vi "lidar_array.vi"(0 "LiDAR Configuration":string="{\n\t\"type\": \"LidarArray\",\n\t\"listen_port\": 6699,\n\t\"location\": {\n\t\t\"x\": 150.0,\n\t\t\"y\": 0.0,\n\t\t\"z\": 60.0\n\t},\n\t\"rotation\": {\n\t\t\"pitch\": 0.0,\n\t\t\"roll\": 0.0,\n\t\t\"yaw\": 0.0\n\t},\n\t\"udp_streamer\": {\n\t\t\"destination_ip\": \"127.0.0.1\",\n\t\t\"udp_packetizer\": \"RSM1\",\n\t\t\"use_udp_streaming\": true\n\t},\n\t\"num_threads\": 10,\n\t\"receive_stream\": false,\n\t\"enable_streaming\": true,\n\t\"firing_data_file_path\":\"\",\n\t\"beam_divergence_horizontal\": 0.009999999776482582,\n\t\"beam_divergence_vertical\": 0.009999999776482582,\n\t\"beam_size_horizontal\": 1.0,\n\t\"beam_size_vertical\": 1.0,\n\t\"debug_draw\": false,\n\t\"diffuse_gain\": 1.0,\n\t\"distance_error\": 1.0,\n\t\"dropout_threshold\": 0.0,\n\t\"intensity_error\": 0.05000000074505806,\n\t\"max_distance\": 150000.0,\n\t\"post_gain\": 1.0,\n\t\"specular_gain\": 1.0,\n\t\"wait_for_fresh_frame\": true,\n\t\"wind_effect\": 0.0\n}", 3 "error in":errorcluster={"status"=FALSE, "code"=0, "source"="\"complete\","}) -> (4 "LiDAR Configuration":string="{\n    \"type\": \"LidarArray\",\n    \"packet_size\": 1472,\n    \"listen_port\": 8201,\n    \"synchronized_display\": true,\n    \"location\": {\n      \"x\": 150.0,\n      \"y\": 0.0,\n      \"z\": 190.0\n    },\n    \"rotation\": {\n      \"pitch\": 0.0,\n      \"yaw\": 0.0,\n      \"roll\": 0.0\n    },\n    \"max_distance\": 10000.0,\n    \"beam_divergence_horizontal\": 0.01,\n    \"beam_divergence_vertical\": 0.01,\n    \"beam_size_horizontal\": 1.0,\n    \"beam_size_vertical\": 1.0,\n    \"distance_error\": 0.075,\n    \"num_threads\": 6,\n    \"intensity_error\": 0.1,\n    \"debug_draw\": false,\n    \"lidar_model\": 0,\n    \"specular_gain\": 1.25,\n    \"diffuse_gain\": 0.95,\n    \"post_gain\": 1.15\n}", 5 "LiDAR Data":T1(array[cluster]), 6 "Raw data":string, 7 "error out":errorcluster={"status"=FALSE, "code"=0, "source"="\"complete\","})   [LabVIEW 2019, in "Lib_Simx.lvlib"]
doc: "Configure and process the data stream for an array LiDAR sensor."
uses:
  Lib_Simx.lvlib
  tools/simx_common.vi
  controls/Header.ctl
panel:
  out "Header":T2
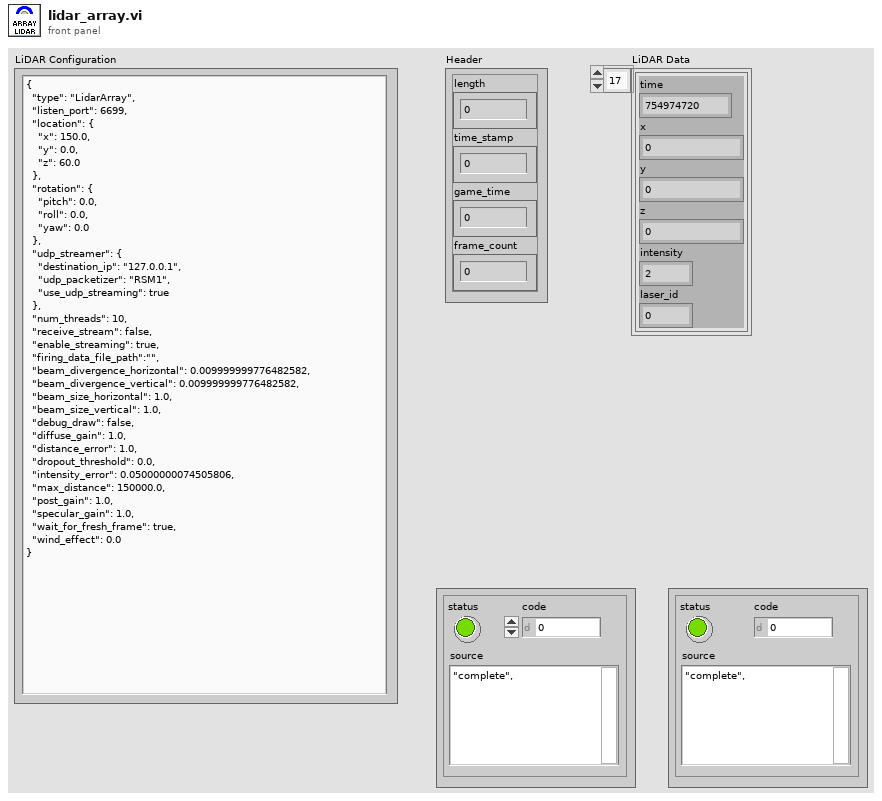
[diagram p1: front panel]
types:
  T1 = cluster{"time":u32, "x":sgl, "y":sgl, "z":sgl, "intensity":u8, "laser_id":u8}[]
  T2 = typedef "Lib_Simx.lvlib/Header.ctl" = cluster{"length":u32, "time_stamp":u32, "game_time":sgl, "frame_count":u32}
  T3 = enum16{"big-endian, network order", "native, host order", "little-endian"}
  T4 = typedef "Lib_Simx.lvlib/sensor_sample.ctl" = cluster{"Header":T2, "data out":string}
  T5 = typedef "Lib_Simx.lvlib/simx_connection.ctl" = cluster{"Config":T6, "Connections":T9, "Map":cluster{"lanes":cluster{"x":dbl[], "y":dbl[], "z":dbl[]}, "StartPosition":cluster{"start_points":T10, "StartRotation":dbl[], "StartLocation":dbl[]}, "Draw Map Size":T11, "DrawArea":cluster{"min_Y":dbl, "min_X":dbl, "Scale X":dbl, "Scale Y":dbl}, "Map":picture, "Map Geojson":string}}
  T6 = typedef "Lib_Simx.lvlib/config.ctl" = cluster{"Trajectory":T7, "Weather":T8}
  T7 = typedef "Lib_Simx.lvlib/trajectory.ctl" = cluster{"Number of frames":i32, "Frame number":i32, "Trajectory":string}
  T8 = typedef "Lib_Simx.lvlib/weather.ctl" = cluster{"id":string}
  T9 = typedef "Lib_Simx.lvlib/connections.ctl" = cluster{"Simulator Connection":refnum<k5>, "server_ip":string, "Port":i32, "Sensor connections":refnum<k5>[]}
  T10 = typedef "Lib_Simx.lvlib/start_points.ctl" = cluster{"locations":dbl[][], "rotations":dbl[][], "type":string[]}
  T11 = typedef "LVBoundsTypeDef.ctl" = cluster{"Width":u32, "Height":u32}
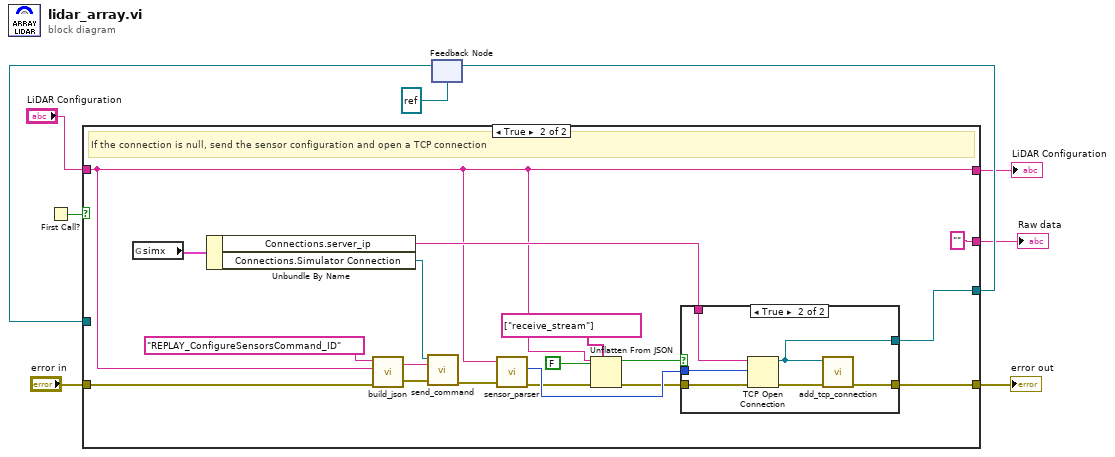
[diagram p0: block diagram]
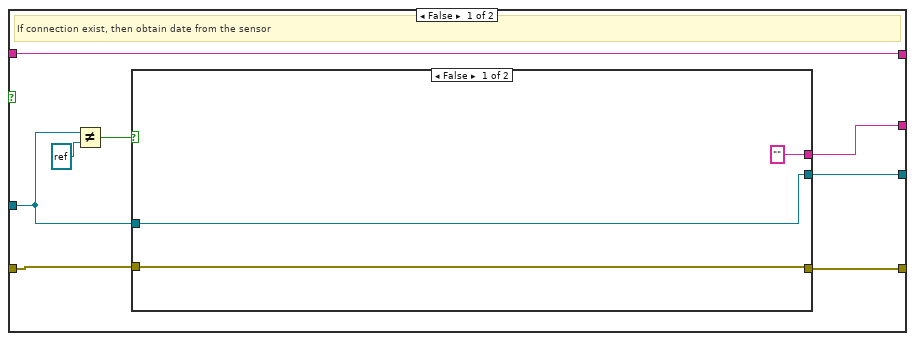
[diagram p2: hidden frame]
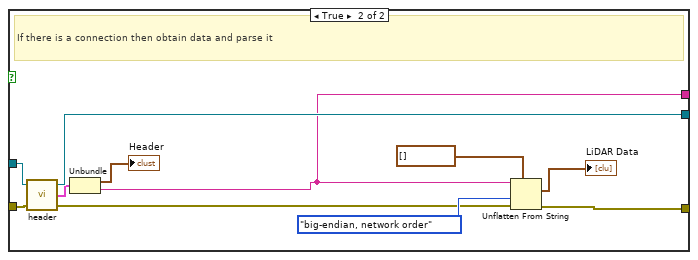
[diagram p3: hidden frame]
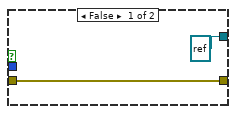
[diagram p4: hidden frame]
diagram:
  n1 = First Call?() -> (First Call?: T/F=w1:bool)
  n2 = feedback #1(refnum<k5> refnum ("lidar_connection")) -> (w5:refnum<k5>)
  n3 = case shown="True" w1 {
    tunnel: [w14 w39] -> w9
    tunnel: "LiDAR Configuration" -> [w15 w36]
    tunnel: [w17 w38] -> w7
    tunnel: w5 -> [w12 _]
    tunnel: "error in" -> [w16 w46]
    tunnel: [w15 w36] -> w3
    tunnel: [w13 "" ("data out")] -> w2
    frame False {
      # "If connection exist, then obtain date from the sensor"
      n4 = Not Equal?(x=w12, y=refnum<k5> refnum) -> (x != y?=w10:bool)
      n5 = case shown="False" w10 {
        tunnel: [w19 w31] -> w17
        tunnel: w16 -> [w20 w30]
        tunnel: [w20 w29] -> w14
        tunnel: ["" ("data out") w28] -> w13
        tunnel: w12 -> [w19 w27]
        frame False {
        }
        frame True {
          # "If there is a connection then obtain data and parse it"
          n6 = call "header.vi"("error in"=w30, "TCP Network Connection in"=w27) -> ("error out"=w22:errorcluster, "Sensor sample"=w26:T4, "TCP Network Connection out"=w31:refnum<k5>)  [unwired: 1 in]
          n7 = Unbundle(w26) -> ("Header"=→"Header":T2, "data out"=w28:string)
          n8 = Unflatten From String(type=T1 [] ("rsm1 format"), binary string=w28, byte order (0:big-endian, network order)=T3."big-endian, network order", error in (no error)=w22) -> (value=→"LiDAR Data":T1, error out=w29:errorcluster)  [unwired: 1 in, 1 out]
        }
      }
    }
    frame True {
      # "If the connection is null, send the sensor configuration and open a TCP connection"
      n9 = global read "simx_common.vi" "simx"() -> (w44:T5)
      n10 = Unbundle By Name(w44) -> ("Connections.server_ip"=w40:string, "Connections.Simulator Connection"=w45:refnum<k5>)
      n11 = call "build_json.vi"("error in"=w46, "Message"=w36, "Command_ID"="REPLAY_ConfigureSensorsCommand_ID") -> ("error out"=w47:errorcluster, "JSON Out"=w48:string)  [unwired: 1 in]
      n12 = call "send_command.vi"("error in"=w47, "JSON Command"=w48, "TCP Network Connection in"=w45) -> ("error out"=w41:errorcluster)  [unwired: 1 in, 3 out]
      n13 = call "sensor_parser.vi"("Sensor configuration"=w36, "error in"=w41) -> ("Port out"=w42:u16, "error out"=w33:errorcluster)  [unwired: 1 in, 2 out]
      n14 = Unflatten From JSON(path=string[] ["receive_stream"], JSON string=w36, type and defaults=FALSE, error in (no error)=w33) -> (value=w35:bool, error out=w32:errorcluster)  [unwired: 3 in]
      n15 = case shown="True" w35 {
        tunnel: w32 -> [w51 w56]
        tunnel: w42 -> [_ w55]
        tunnel: w40 -> [_ w54]
        tunnel: [w51 w53] -> w39
        tunnel: [refnum<k5> refnum ("connection ID") w52] -> w38
        frame False {
        }
        frame True {
          n16 = TCP Open Connection(address=w54, remote port or service name=w55, error in (no error)=w56) -> (connection ID=w52:refnum<k5>, error out=w57:errorcluster)  [unwired: 2 in]
          n17 = call "add_tcp_connection.vi"("error in"=w57, "Sensor connection"=w52) -> ("error out"=w53:errorcluster)  [unwired: 5 in]
        }
      }
    }
  }
  "error out" <- w9
  "LiDAR Configuration" <- w3
  "Raw data" <- w2
  n18 = feedback-in #1(w7) -> ()
